vi "#21_MAV_MSG_PARAM_REQUEST_LIST_ENCODE.vi"(10 "packet_sequence_in":u8, 11 "PARAM_REQUEST_LIST":T1={"self"={"system_id"=255, "component_id"=190}, "target_system_id"=0, "target_component_id"=0}) -> (2 "packet_sequence_out":u8, 3 "mavlink_buffer_out":u8[](array[numeric]))   [LabVIEW 2023]
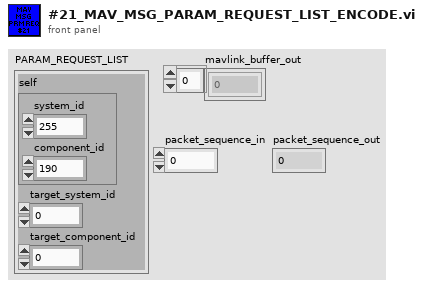
[diagram p1: front panel]
types:
  T1 = cluster{"self":cluster{"system_id":u8, "component_id":u8}, "target_system_id":u8, "target_component_id":u8}
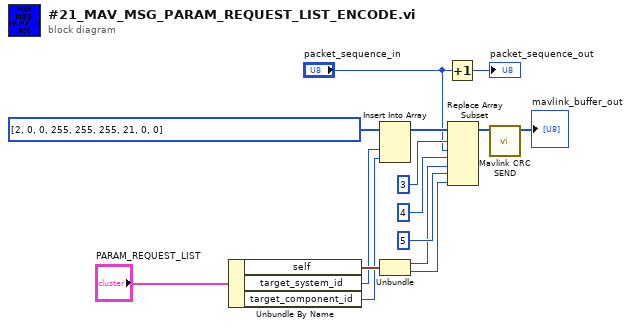
[diagram p0: block diagram]
diagram:
  n1 = Unbundle By Name("PARAM_REQUEST_LIST") -> ("self"=w12:cluster{"system_id":u8, "component_id":u8}, "target_system_id"=w11:u8, "target_component_id"=w10:u8)
  n2 = Insert Into Array(array=u8[] [2, 0, 0, 255, 255, 255, 21, 0, 0], new element #1=w11, new element #2=w10) -> (w9:u8[])  [unwired: 1 in]
  n3 = Unbundle(w12) -> ("system_id"=w4:u8, "component_id"=w3:u8)
  n4 = Increment(x="packet_sequence_in") -> (x+1=→"packet_sequence_out":u8)
  n5 = Replace Array Subset(array=w9, new element #1="packet_sequence_in", index #1=3 ("index"), new element #2=w4, index #2=4 ("index"), new element #3=w3, index #3=5 ("index")) -> (w2:u8[])
  n6 = call "Mavlink CRC SEND.vi"("Byte In"=w2) -> ("Output Byte"=→"mavlink_buffer_out":u8[])  [unwired: 10 in]
